vi "Log Value to File.vi"(8 "error in (no error)":errorcluster, 10 "Data Record":T1, 11 "Datalogger object in":refnum<class "Datalogger.lvclass">) -> (0 "error out":errorcluster, 3 "Datalogger object out":refnum<class "Datalogger.lvclass">)   [LabVIEW 2018, in "Datalogger.lvlib" / "Datalogger.lvclass"]
uses:
  Datalogger.lvclass
  Data Record Control.ctl
  Datalogger.lvclass/Datalogger.ctl
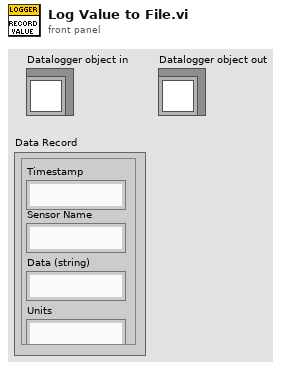
[diagram p1: front panel]
types:
  T1 = typedef "Datalogger.lvlib/Datalogger.lvclass/Data Record Control.ctl" = cluster{"Timestamp":string, "Sensor Name":string, "Data (string)":string, "Units":string}
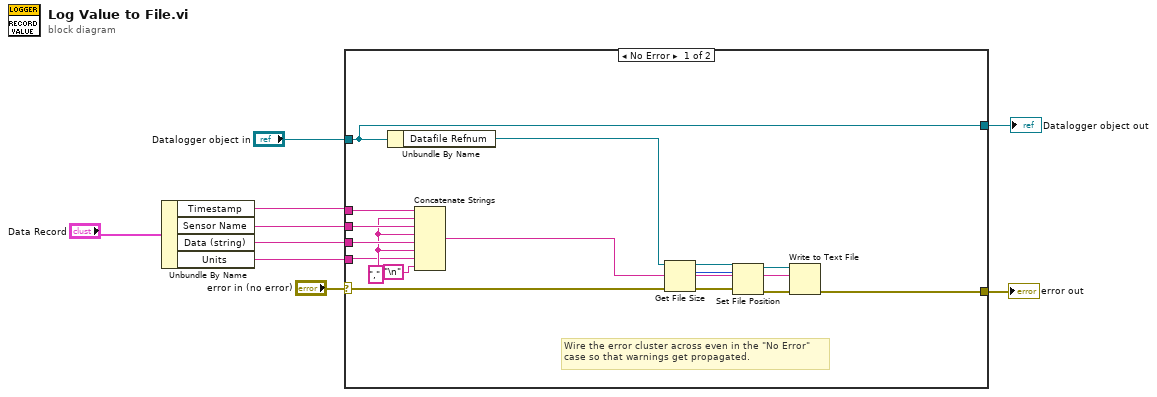
[diagram p0: block diagram]
diagram:
  n1 = Unbundle By Name("Data Record") -> ("Timestamp"=w5:string, "Sensor Name"=w4:string, "Data (string)"=w7:string, "Units"=w6:string)
  n2 = case shown="No Error" "error in (no error)" {
    selector: "error in (no error)" -> [w18 w27]
    tunnel: [w25 w27] -> w8
    tunnel: w7 -> [w22 _]
    tunnel: w6 -> [w19 _]
    tunnel: w5 -> [w24 _]
    tunnel: w4 -> [w23 _]
    tunnel: "Datalogger object in" -> [w10 w26]
    tunnel: [w10 w26] -> w2
    frame No Error {
      w21 = "," ("string")
      # "Wire the error cluster across even in the \"No Error\"\ncase so that warnings get propagated."
      n3 = Unbundle By Name(w10) -> ("Datafile Refnum"=w11:refnum<file>)
      n4 = Concatenate Strings(w24, w21, w23, w21, w22, w21, w19, "\n") -> (w13:string)
      n5 = Get File Size(file=w11, error in=w18) -> (refnum out=w17:refnum<file>, size (in bytes)=w12:i64, 0:w15:errorcluster)
      n6 = Set File Position(offset (in bytes) (0)=w12, refnum=w17, error in=w15) -> (refnum out=w16:refnum<file>, error out=w14:errorcluster)  [unwired: 1 in]
      n7 = Write to Text File(file (use dialog)=w16, text=w13, error in=w14) -> (error out=w25:errorcluster)  [unwired: 1 in, 2 out]
    }
    frame Error {
    }
  }
  "error out" <- w8
  "Datalogger object out" <- w2
